vi "Fluke 6105A Flicker Set.vi"() -> ()   [LabVIEW 2014]
doc: "This example shows how to configure and use all noise features on a single output."
uses:
  SharedVariables/TSE_Variables.vi
panel:
  in  "RMS":i32
  in  "Fluct or Flick":enum32{"Flicker"}(tab)
  in  "Frequency":dbl=40.0
  in  "Depth":dbl=60.0
  in  "Duty Cycle":dbl=15.0
  in  "Shape":string(combo)="SQU"
  in  "Enable Flicker?":bool
  in  "Harmonics":cluster{"Amplitude":dbl, "Phase Angle":dbl}[](array[cluster])=[{"Amplitude"=10.0, "Phase Angle"=0.0}, {"Amplitude"=120.0, "Phase Angle"=0.0}, {"Amplitude"=0.0, "Phase Angle"=0.0}, {"Amplitude"=0.0, "Phase Angle"=0.0}, {"Amplitude"=0.0, "Phase Angle"=0.0}, {"Amplitude"=20.0, "Phase Angle"=0.0}, {"Amplitude"=0.0, "Phase Angle"=0.0}, {"Amplitude"=0.0, "Phase Angle"=0.0}, {"Amplitude"=0.0, "Phase Angle"=0.0}, {"Amplitude"=35.0, "Phase Angle"=56.0}]
  in  "Upper Range (2)":dbl=250.0
  in  "Lower Range (1)":dbl=100.0
  in  "Voltage or Current":enum16{"Voltage", "Current"}(ring)
  in  "Output Selector":u16(ring)=1 items=["L1"=1, "L2"=2, "L3"=3, "N"=4]
  in  "Enable Harmonics?":bool=TRUE
  in  "Sense Setting (1:4-wire)":u16(ring)=1 items=["2-wire sensing", "4-wire sensing"]
  in  "Line Locking":bool
  in  "Angle Setting (0: Degrees)":string(combo)="DEG"
  in  "Current Harmonics Amplitude":string(combo)="ABS"
  in  "Voltage Harmonics Amplitude":string(combo)="ABS"
  in  "Frequency (Hz)":i32=60
  in  "stop":bool
  in  "VISA resource name":refnum<visa-resource-name>
  # "(c) 2004 - 2010 National Instruments.  ALL RIGHTS RESERVED."
  # "Harmonics"
  # "Global Settings"
  # "Note: The RMS value is only set\nwhen the Harmonics Amplitude\nmode is \"% of RMS\""
  # "Flicker"
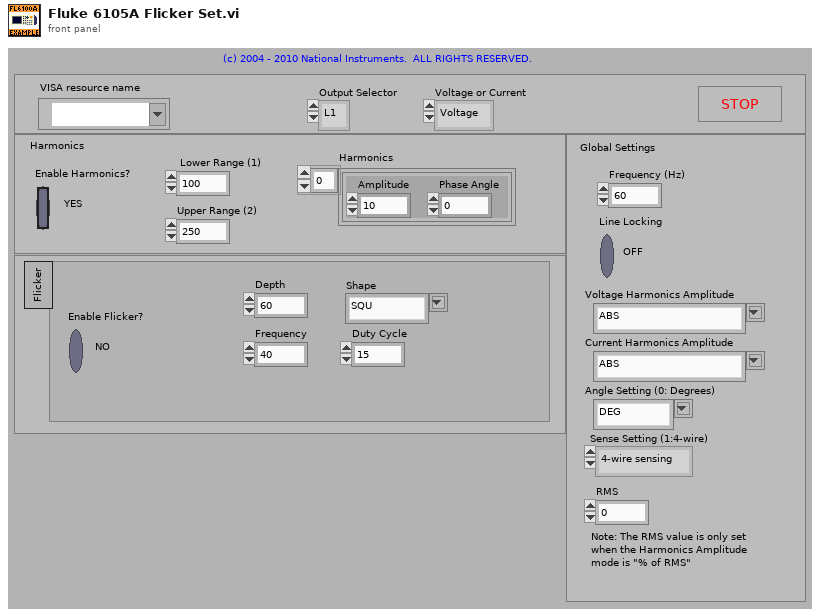
[diagram p1: front panel]
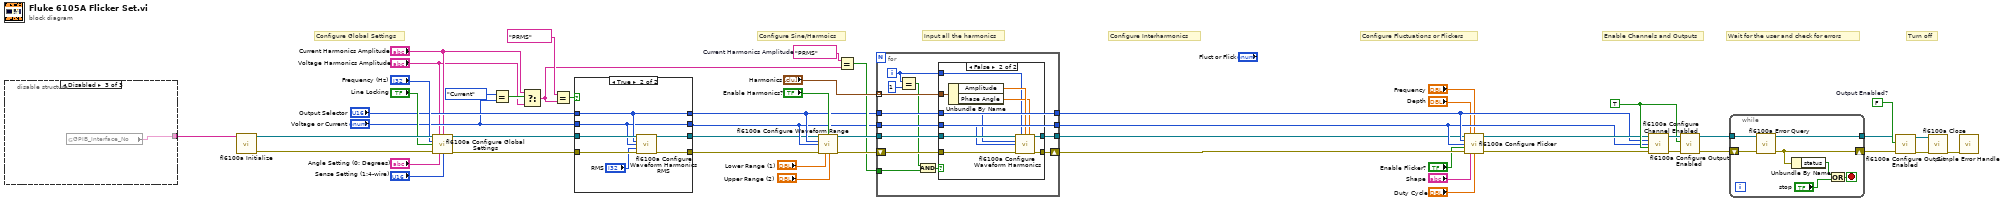
[diagram p0: block diagram]
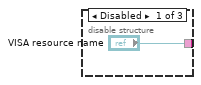
[diagram p2: hidden frame]
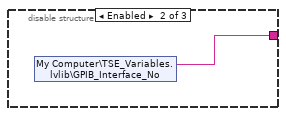
[diagram p3: hidden frame]
diagram:
  w13 = "PRMS"  # Current Harmonics Amplitude
  w45 = FALSE  # Output Enabled?
  w29 = TRUE ("Output Enabled? (F:Off)")
  # "Turn off"
  # "Wait for the user and check for errors"
  # "Enable Channels and Outputs"
  # "Configure Fluctuations or Flickers"
  # "Configure Interharmonics"
  # "Input all the harmonics"
  # "Configure Sine/Harmoics"
  # "Configure Global Settings"
  n1 = disable-structure shown="Disabled" {
    disable-tunnel: ["VISA resource name" w54 w55] -> w52
    frame Disabled {
    }
    frame Enabled {
      n2 = shared-variable "My Computer\\TSE_Variables.lvlib\\GPIB_Interface_No"() -> (w54:string)  [unwired: 1 in, 1 out]
    }
    frame Disabled {
      n3 = global read "TSE_Variables.vi" "GPIB_Interface_No"() -> (w55:string)
    }
  }
  n4 = call <instrlib>:"fl6100a Initialize.vi"("VISA resource name"=w52) -> ("error out"=w50:errorcluster, "VISA resource name out"=w51:refnum<visa-resource-name>)  [unwired: 9 in]
  n5 = call <instrlib>:"fl6100a Configure Global Settings.vi"("VISA resource name"=w51, "Voltage Harmonics Amplitude (0: Absolute RMS)"="Voltage Harmonics Amplitude", "Current Harmonics Amplitude (0: Absolute RMS)"="Current Harmonics Amplitude", "Frequency (60 Hz)"="Frequency (Hz)", "Line Locking (F: Off)"="Line Locking", "error in (no error)"=w50, "Angle Setting (0: Degrees)"="Angle Setting (0: Degrees)", "Sense Setting (1:4-wire)"="Sense Setting (1:4-wire)") -> ("VISA resource name out"=w24:refnum<visa-resource-name>, "error out"=w23:errorcluster)  [unwired: 6 in]
  n6 = Equal?(x=enum16{"Voltage", "Current"}."Current", y="Voltage or Current") -> (x = y?=w19:bool)
  n7 = Select(t="Current Harmonics Amplitude", s=w19, f="Voltage Harmonics Amplitude") -> (s? t:f=w14:string)
  n8 = Equal?(x="PRMS" ("Current Harmonics Amplitude"), y=w14) -> (x = y?=w16:bool)
  n9 = case shown="True" w16 {
    tunnel: w24 -> [w57 w66]
    tunnel: w23 -> [w56 w65]
    tunnel: [w57 w64] -> w9
    tunnel: [w56 w63] -> w8
    tunnel: "Output Selector" -> [w59 w61]
    tunnel: "Voltage or Current" -> [w58 w60]
    tunnel: [w59 w61] -> w11
    tunnel: [w58 w60] -> w10
    frame False {
    }
    frame True {
      n10 = call <instrlib>:"fl6100a Configure Waveform Harmonics RMS.vi"("VISA resource name"=w66, "Output Selector (0:L1)"=w61, "Voltage or Current (0: Voltage)"=w60, "RMS (0)"="RMS", "error in (no error)"=w65) -> ("VISA resource name out"=w64:refnum<visa-resource-name>, "error out"=w63:errorcluster)  [unwired: 9 in]
    }
  }
  n11 = call <instrlib>:"fl6100a Configure Waveform Range.vi"("VISA resource name"=w9, "Enable Equivalence Factor (Y:YES)"="Enable Harmonics?", "Output Selector (0:L1)"=w11, "Voltage or Current (0: Voltage)"=w10, "error in (no error)"=w8, "Lower Range (1)"="Lower Range (1)", "Upper Range (2)"="Upper Range (2)") -> ("VISA resource name out"=w32:refnum<visa-resource-name>, "error out"=w31:errorcluster)  [unwired: 7 in]
  n12 = Equal?(x=w13, y=w14) -> (x = y?=w12:bool)
  n13 = for {
    tunnel: [w78] -> w7
    tunnel: w32 -> [w76]
    tunnel: w11 -> [w73]
    tunnel: w10 -> [w72]
    tunnel: "Harmonics" -> [w74] mode=indexing
    tunnel: [w73] -> w26
    tunnel: [w72] -> w25
    shift-right: [w77] -> w6
    shift-left: w31 -> [w75]
    tunnel: w12 -> [w68]
    i -> [w71]
    n14 = Equal?(x=w71, y=1) -> (x = y?=w69:bool)
    n15 = And(x=w69, y=w68) -> (x .and. y?=w70:bool)
    n16 = case shown="False" w70 {
      tunnel: [w80 w90] -> w78
      tunnel: [w79 w89] -> w77
      tunnel: w76 -> [w80 w88]
      tunnel: w75 -> [w79 w87]
      tunnel: w74 -> [_ w86]
      tunnel: w73 -> [_ w83]
      tunnel: w72 -> [_ w82]
      tunnel: w71 -> [_ w81]
      frame True {
      }
      frame False {
        n17 = Unbundle By Name(w86) -> ("Amplitude"=w85:dbl, "Phase Angle"=w84:dbl)
        n18 = call <instrlib>:"fl6100a Configure Waveform Harmonics.vi"("VISA resource name"=w88, "Harmonic (1)"=w81, "Amplitude (1)"=w85, "Phase Angle (0)"=w84, "Output Selector (0:L1)"=w83, "Voltage or Current (0: Voltage)"=w82, "error in (no error)"=w87) -> ("VISA resource name out"=w90:refnum<visa-resource-name>, "error out"=w89:errorcluster)  [unwired: 7 in]
      }
    }
  }
  n19 = call <instrlib>:"fl6100a Configure Flicker.vi"("VISA resource name"=w7, "Flicker Depth (0 %)"="Depth", "Flicker Frequency (13.5 Hz)"="Frequency", "Output Selector (0:L1)"=w26, "Voltage or Current (0: Voltage)"=w25, "Enable Flicker? (F:NO)"="Enable Flicker?", "error in (no error)"=w6, "Flicker Shape (Sinusoidal)"="Shape", "Flicker Duty Cycle (0 %)"="Duty Cycle") -> ("VISA resource name out"=w28:refnum<visa-resource-name>, "error out"=w27:errorcluster)  [unwired: 5 in]
  n20 = call <instrlib>:"fl6100a Configure Channel Enabled.vi"("VISA resource name"=w28, "Output Selector (0:L1)"=w26, "Voltage or Current (0: Voltage)"=w25, "Enable Channel? (F:NO)"=w29, "error in (no error)"=w27) -> ("VISA resource name out"=w49:refnum<visa-resource-name>, "error out"=w48:errorcluster)  [unwired: 9 in]
  n21 = call <instrlib>:"fl6100a Configure Output Enabled.vi"("error in (no error)"=w48, "Enable Output? (F:NO)"=w29, "VISA resource name"=w49) -> ("error out"=w46:errorcluster, "VISA resource name out"=w47:refnum<visa-resource-name>)  [unwired: 7 in]
  n22 = while {
    tunnel: w47 -> [w97]
    tunnel: [w95] -> w44
    shift-right: [w94] -> w43
    shift-left: w46 -> [w96]
    stop <- w93 stop-if-true
    n23 = call <instrlib>:"fl6100a Error Query.vi"("error in (no error)"=w96, "VISA resource name"=w97) -> ("error out"=w94:errorcluster, "VISA resource name out"=w95:refnum<visa-resource-name>)  [unwired: 6 in, 2 out]
    n24 = Unbundle By Name(w94) -> ("status"=w92:bool)
    n25 = Or(x=w92, y="stop") -> (x .or. y?=w93:bool)
  }
  n26 = call <instrlib>:"fl6100a Configure Output Enabled.vi"("error in (no error)"=w43, "Enable Output? (F:NO)"=w45, "VISA resource name"=w44) -> ("error out"=w41:errorcluster, "VISA resource name out"=w42:refnum<visa-resource-name>)  [unwired: 7 in]
  n27 = call <instrlib>:"fl6100a Close.vi"("error in (no error)"=w41, "VISA resource name"=w42) -> ("error out"=w40:errorcluster)  [unwired: 9 in]
  n28 = call <vilib>:"Simple Error Handler.vi"("error in (no error)"=w40) -> ()  [unwired: 4 in, 5 out]
